vi "Read Characters From File with Options.vi"(0 "file path (dialog if empty)":path, 1 "prompt":string="Choose file to read.", 5 "start path (Not A Path)":path=path "", 7 "default name":string, 9 "[pattern]":string, 11 "number of characters (all:-1)":i32=-1, 12 "convert eol? (no:F)":bool, 13 "start of read offset (chars.: 0)":i32) -> (4 "new file path (NotAPath if cancelled)":path, 6 "character string":string, 8 "mark after read (chars.)":i32, 10 "EOF?":bool, 15 "error out":errorcluster)   [LabVIEW 2023]
doc: "Reads a specified number of characters from a byte stream file beginning at a specified character offset."
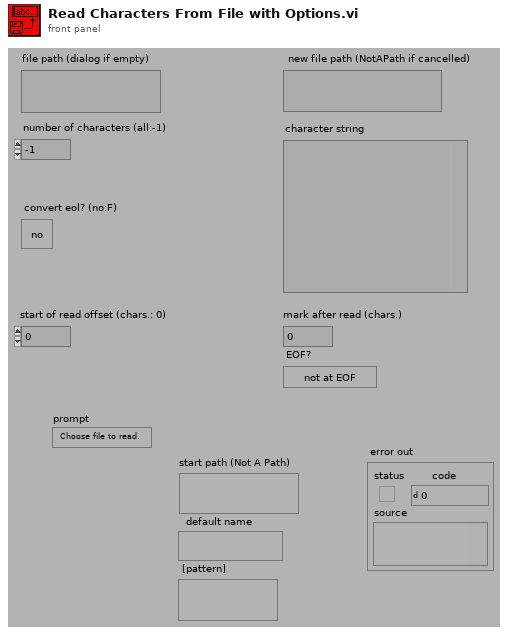
[diagram p1: front panel]
types:
  T1 = enum16{"read/write", "read-only", "write-only", "write-only (truncate)"}
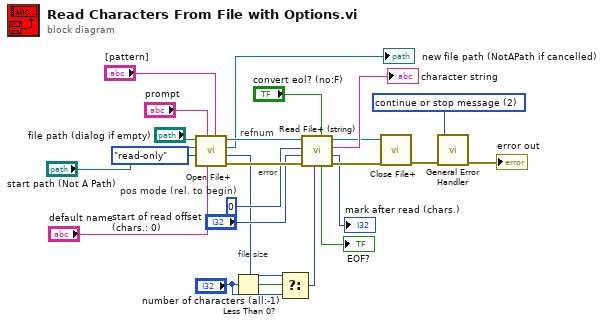
[diagram p0: block diagram]
diagram:
  w1 = u16 2 items=["no dialog", "OK message", "continue or stop message"] ("type of dialog (OK msg:1)")
  w21 = i16 0  # pos mode (rel. to begin)
  # "file size"
  # "error"
  # "refnum"
  n1 = call <vilib>:"Open File+.vi"("[pattern]"="[pattern]", "default name"="default name", "prompt"="prompt", "open mode (read-only:1)"=T1."read-only", "start path (Not A Path)"="start path (Not A Path)", "file path (\" \")"="file path (dialog if empty)") -> ("error out"=w23:errorcluster, "file size (bytes)"=w12:i32, "file path"=→"new file path (NotAPath if cancelled)":path, "refnum"=w15:refnum<file>)  [unwired: 2 in]
  n2 = Less Than 0?(x="number of characters (all:-1)") -> (x < 0?=w13:bool)
  n3 = Select(t=w12, s=w13, f="number of characters (all:-1)") -> (s? t:f=w10:i32)
  n4 = call <vilib>:"Read File+ (string).vi"("convert eol? (no:F)"="convert eol? (no:F)", "count"=w10, "error in (no error)"=w23, "pos offset (bytes:0)"="start of read offset (chars.: 0)", "pos mode (rel. to current:2)"=w21, "refnum"=w15) -> ("error out"=w19:errorcluster, "mark after read (bytes)"=→"mark after read (chars.)":i32, "string"=→"character string":string, "dup refnum"=w18:refnum<file>, "EOF?"=→"EOF?":bool)  [unwired: 1 in]
  n5 = call <vilib>:"Close File+.vi"("error in (no error)"=w19, "refnum"=w18) -> ("error out"=w2:errorcluster)  [unwired: 3 in, 2 out]
  n6 = call <vilib>:"General Error Handler.vi"("type of dialog (OK msg:1)"=w1, "error in (no error)"=w2) -> ("error out"=→"error out":errorcluster)  [unwired: 9 in, 4 out]
